vi "Memory.Pointer.Swap.Safe.vi"(8 "error in (no error)":errorcluster, 10 "pointer b":refnum<class "Memory.Pointer.lvclass">, 11 "pointer a":refnum<class "Memory.Pointer.lvclass">) -> (0 "error out":errorcluster, 2 "pointer b":refnum<class "Memory.Pointer.lvclass">, 3 "pointer a":refnum<class "Memory.Pointer.lvclass">)   [LabVIEW 2016, in "Memory.lvlib" / "Memory.Pointer.lvclass"]
doc: "Swaps the address of the two provided <b>pointers</b>. This cannot be used with external pointers created via the Encapsulate method.\n\n<b>Note:</b> This VI is <b>safe</b>.\n\nSafe means that this function evaluates the size parameter of <b>pointer a</b> and <b>pointer b</b> to ensure that the memory location associated with each pointer is the same size before peforming a memory read/write. Reading/writing more data to a pointer than it has allocated can corrupt or crash LabVIEW."
uses:
  Memory.Pointer.lvclass
  Memory.Pointer.lvclass/Memory.Pointer.ctl
  Memory.Pointer.Errors.Size Mismatch.vi
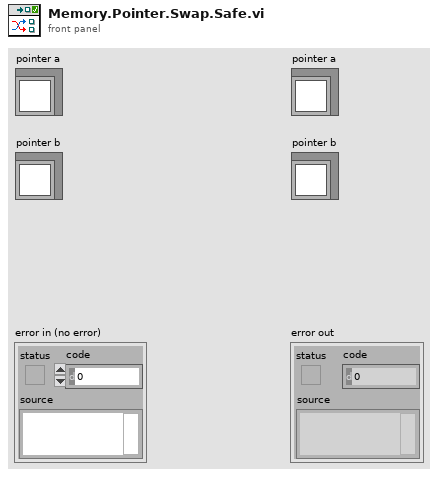
[diagram p1: front panel]
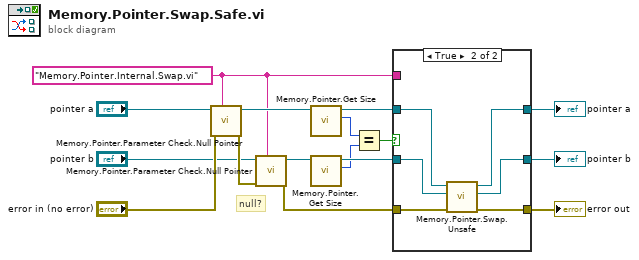
[diagram p0: block diagram]
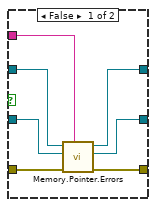
[diagram p2: hidden frame]
diagram:
  w1 = "Memory.Pointer.Internal.Swap.vi" ("source vi name")
  # "null?"
  n1 = call "Memory.Pointer.Parameter Check.Null Pointer.vi"("source vi name"=w1, "error in (no error)"="error in (no error)", "Pointer in"="pointer a") -> ("error out"=w5:errorcluster, "Pointer out"=w7:refnum<class "Memory.Pointer.lvclass">)  [unwired: 7 in]
  n2 = call "Memory.Pointer.Parameter Check.Null Pointer.vi"("source vi name"=w1, "error in (no error)"=w5, "Pointer in"="pointer b") -> ("error out"=w3:errorcluster, "Pointer out"=w6:refnum<class "Memory.Pointer.lvclass">)  [unwired: 7 in]
  n3 = call "Memory.Pointer.Get Size.vi"("Pointer in"=w7) -> ("size"=w10:u64, "Pointer out"=w15:refnum<class "Memory.Pointer.lvclass">)  [unwired: 9 in]
  n4 = call "Memory.Pointer.Get Size.vi"("Pointer in"=w6) -> ("size"=w9:u64, "Pointer out"=w14:refnum<class "Memory.Pointer.lvclass">)  [unwired: 9 in]
  n5 = Equal?(x=w10, y=w9) -> (x = y?=w16:bool)
  n6 = case shown="True" w16 {
    tunnel: w15 -> [w21 w25]
    tunnel: w14 -> [w19 w29]
    tunnel: [w20 w24] -> w13
    tunnel: [w18 w28] -> w12
    tunnel: w3 -> [w23 w27]
    tunnel: [w22 w26] -> w11
    tunnel: w1 -> [w17 _]
    frame False {
      n7 = call-poly "Memory.Pointer.Errors.vi"("source vi name"=w17, "error in (no error)"=w23, "pointer b in"=w19, "pointer a in"=w21) -> ("error out"=w22:errorcluster, "pointer b out"=w18:refnum<class "Memory.Pointer.lvclass">, "pointer a out"=w20:refnum<class "Memory.Pointer.lvclass">)  [unwired: 5 in]
    }
    frame True {
      n8 = call "Memory.Pointer.Swap.Unsafe.vi"("error in (no error)"=w27, "pointer b"=w29, "pointer a"=w25) -> ("error out"=w26:errorcluster, "pointer b"=w28:refnum<class "Memory.Pointer.lvclass">, "pointer a"=w24:refnum<class "Memory.Pointer.lvclass">)  [unwired: 6 in]
    }
  }
  "error out" <- w11
  "pointer a" <- w13
  "pointer b" <- w12
